vi "WFComposeCanA.vi"(8 "error in (no error)":errorcluster, 10 "WFRepetitions":T1={"Del (s)"=0.0, "Int (s)"=0.0, "N"=1} {"Int (s)" min=0.0 format="%#_4g"; "Del (s)" min=0.0 format="%#_4f"}, 11 "Waveform In":waveform(dbl)={"t0"=timestamp(0 s since 1904-01-01), "dt"=0.0, "Y"=[]}) -> (0 "error out":errorcluster, 3 "ComposeCan":bool)   [LabVIEW 2013]
doc: "This VI tests whether an input waveform can be composed based on the repetition parameters specified. Implementation function for WFCompose"
uses:
  WFRepetitions.ctl
  <vilib>/Waveform/WDTOps.llb/WDT Waveform Duration DBL.vi
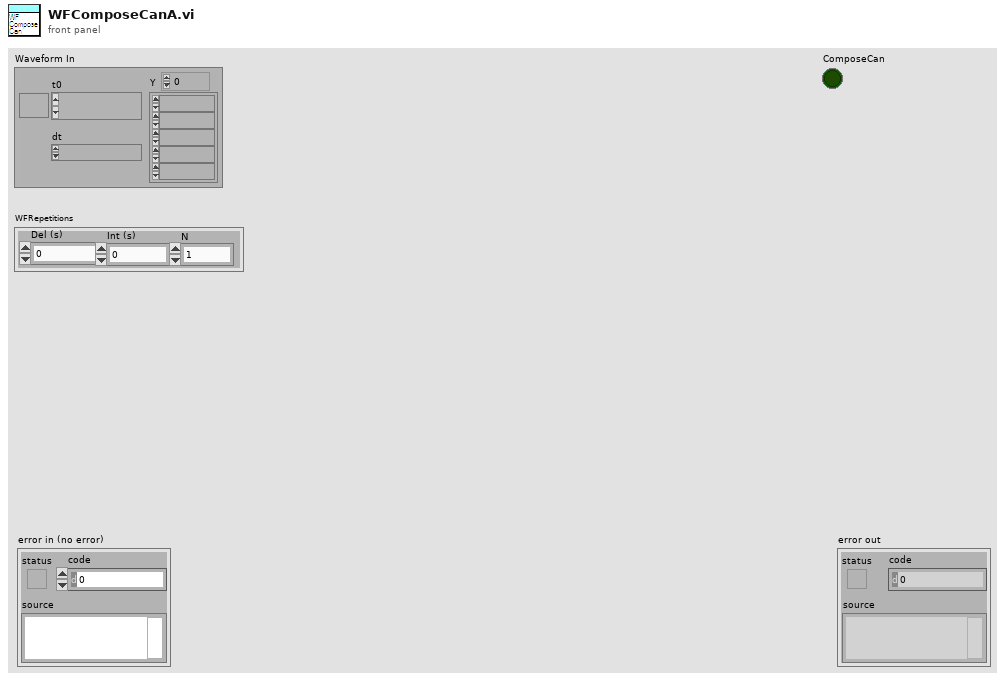
[diagram p1: front panel]
types:
  T1 = typedef "WFRepetitions.ctl" = cluster{"Del (s)":dbl, "Int (s)":dbl, "N":i32}
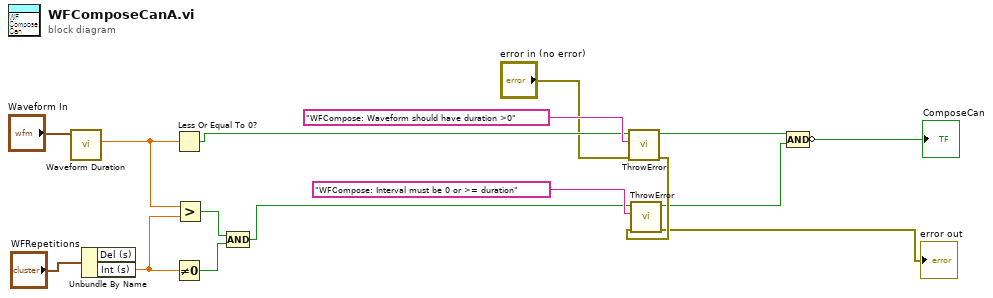
[diagram p0: block diagram]
diagram:
  n1 = call-poly <vilib>:"Waveform Duration.vi"("waveform in"="Waveform In") -> ("duration"=w15:dbl)  [unwired: 8 in, 2 out]
  n2 = Unbundle By Name("WFRepetitions") -> ("Int (s)"=w12:dbl)  [unwired: 1 out]
  n3 = Less Or Equal To 0?(x=w15) -> (x <= 0?=w10:bool)
  n4 = Not Equal To 0?(x=w12) -> (x != 0?=w14:bool)
  n5 = Greater?(x=w15, y=w12) -> (0:w7:bool)
  n6 = Compound Arithmetic op=AND(w7, w14) -> (w6:bool)
  n7 = call "ThrowError.vi"("error in (no error)"="error in (no error)", "Error Message"="WFCompose: Waveform should have duration >0", "Error Input"=w10) -> ("error out"=w4:errorcluster, "Error Input Passthrough"=w9:bool)  [unwired: 7 in]
  n8 = call "ThrowError.vi"("error in (no error)"=w4, "Error Message"="WFCompose: Interval must be 0 or >= duration", "Error Input"=w6) -> ("error out"=→"error out":errorcluster, "Error Input Passthrough"=w2:bool)  [unwired: 7 in]
  n9 = Compound Arithmetic op=AND(w9, w2) -> (invert →"ComposeCan":bool)
